vi "Query Time.vi"(8 "Error In":errorcluster, 11 "NTP Server":string) -> (0 "Error Out":errorcluster, 2 "NTP Packet":T1, 3 "Time Stamp":timestamp)   [LabVIEW 2021, in "SNTP.lvlib"]
uses:
  SNTP.lvlib
  Controls/NTP Packet.ctl
  Controls/Time Stamp 64.ctl
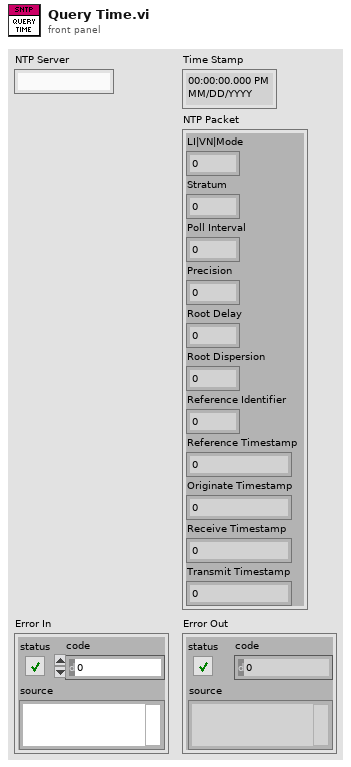
[diagram p1: front panel]
types:
  T1 = typedef "SNTP.lvlib/NTP Packet.ctl" = cluster{"LI|VN|Mode":u8, "Stratum":u8, "Poll Interval":u8, "Precision":i8, "Root Delay":u32, "Root Dispersion":u32, "Reference Identifier":u32, "Reference Timestamp":T2, "Originate Timestamp":T2, "Receive Timestamp":T2, "Transmit Timestamp":T2}
  T2 = typedef "SNTP.lvlib/Time Stamp 64.ctl" = fxp<+,64,32>
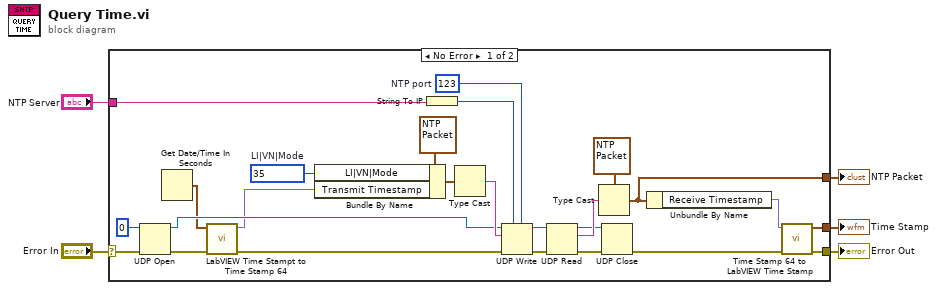
[diagram p0: block diagram]
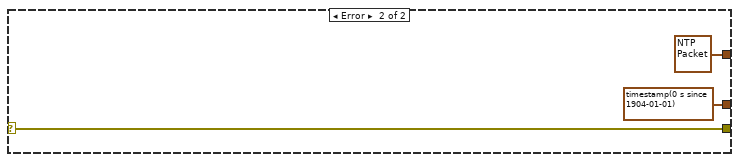
[diagram p2: hidden frame]
diagram:
  n1 = case shown="No Error" "Error In" {
    selector: "Error In" -> [w29 w31]
    tunnel: [w15 T1 {"LI|VN|Mode"=0, "Stratum"=0, "Poll Interval"=0, "Precision"=0, "Root Delay"=0, "Root Dispersion"=0, "Reference Identifier"=0, "Reference Timestamp"=0.0, "Originate Timestamp"=0.0, "Receive Timestamp"=0.0, "Transmit Timestamp"=0.0} ("NTP Packet")] -> w4
    tunnel: [w13 timestamp(0 s since 1904-01-01) ("LabVIEW Time Stamp")] -> w3
    tunnel: [w11 w31] -> w2
    tunnel: "NTP Server" -> [w8 _]
    frame No Error {
      w7 = u16 123  # NTP port
      w28 = u8 35  # LI|VN|Mode
      n2 = UDP Open(8:w29, 11:u16 0 ("port")) -> (port=w19:refnum<k16>, 0:w27:errorcluster)  [unwired: 3 in, 1 out]
      n3 = Get Date/Time In Seconds() -> (seconds since 1Jan1904=w9:timestamp)
      n4 = call "LabVIEW Time Stampt to Time Stamp 64.vi"("Error In"=w27, "LabVIEW Time Stamp"=w9) -> ("Error Out"=w18:errorcluster, "Time Stamp 64"=w17:T2)  [unwired: 8 in]
      n5 = Bundle By Name(cluster=T1 {"LI|VN|Mode"=0, "Stratum"=0, "Poll Interval"=0, "Precision"=0, "Root Delay"=0, "Root Dispersion"=0, "Reference Identifier"=0, "Reference Timestamp"=0.0, "Originate Timestamp"=0.0, "Receive Timestamp"=0.0, "Transmit Timestamp"=0.0} ("NTP Packet"), "LI|VN|Mode"=w28, "Transmit Timestamp"=w17) -> (w25:T1)
      n6 = String To IP(1:w8) -> (0:w10:u32)
      n7 = Type Cast(x=w25) -> (*(type *) &x=w20:string)  [unwired: 1 in]
      n8 = UDP Write(address=w10, port or service name=w7, connection ID=w19, data in=w20, 8:w18) -> (error out=w21:errorcluster, 3:w22:refnum<k16>)  [unwired: 1 in]
      n9 = UDP Read(connection ID=w22, 8:w21) -> (data out=w24:string, error out=w6:errorcluster, 3:w23:refnum<k16>)  [unwired: 2 in, 2 out]
      n10 = Type Cast(type=T1 {"LI|VN|Mode"=0, "Stratum"=0, "Poll Interval"=0, "Precision"=0, "Root Delay"=0, "Root Dispersion"=0, "Reference Identifier"=0, "Reference Timestamp"=0.0, "Originate Timestamp"=0.0, "Receive Timestamp"=0.0, "Transmit Timestamp"=0.0} ("NTP Packet"), x=w24) -> (*(type *) &x=w15:T1)
      n11 = UDP Close(connection ID=w23, 8:w6) -> (error out=w16:errorcluster)  [unwired: 1 out]
      n12 = Unbundle By Name(w15) -> ("Receive Timestamp"=w14:T2)
      n13 = call "Time Stamp 64 to LabVIEW Time Stamp.vi"("Error In"=w16, "Time Stamp 64"=w14) -> ("Error Out"=w11:errorcluster, "LabVIEW Time Stamp"=w13:timestamp)  [unwired: 8 in]
    }
    frame Error {
    }
  }
  "Error Out" <- w2
  "Time Stamp" <- w3
  "NTP Packet" <- w4
